vi "put_chair_cushions.vi"(8 "error in":errorcluster, 11 "chairs in":refnum<class "IChair.lvclass">[](array[class])) -> (0 "error out":errorcluster, 2 "cushion results":string[](array[string]), 3 "chairs out":refnum<class "IChair.lvclass">[](array[class]))   [LabVIEW 2021]
uses:
  IChair/IChair.lvclass
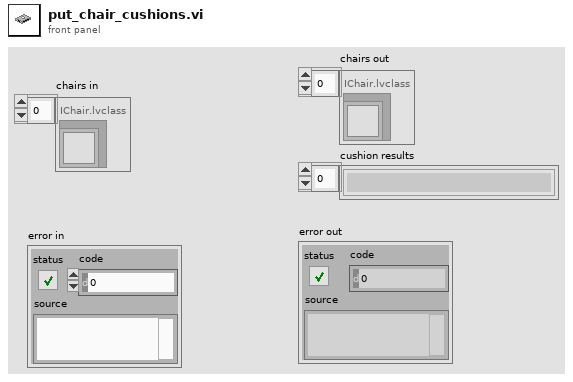
[diagram p1: front panel]
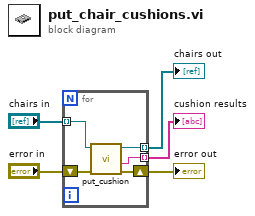
[diagram p0: block diagram]
diagram:
  n1 = for {
    tunnel: "chairs in" -> [w10] mode=indexing
    tunnel: [w9] -> w4 mode=indexing
    tunnel: [w8] -> w3 mode=indexing
    shift-right: [w6] -> w1
    shift-left: "error in" -> [w7]
    n2 = call-dynamic "put_cushion.vi"("error in (no error)"=w7, "IChair.lvclass"=w10) -> ("error out"=w6:errorcluster, "result"=w8:string, "IChair.lvclass"=w9:refnum<class "IChair.lvclass">)  [unwired: 7 in]
  }
  "chairs out" <- w4
  "cushion results" <- w3
  "error out" <- w1
